vi "Test_firmware_propmt.vi"(8 "WIFI Listo":bool, 11 "ESP32 Listo":bool) -> (2 "Resultado":bool)   [LabVIEW 2025]
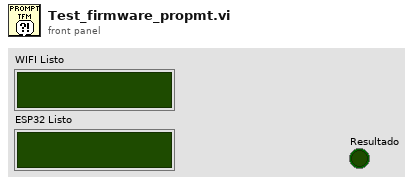
[diagram p1: front panel]
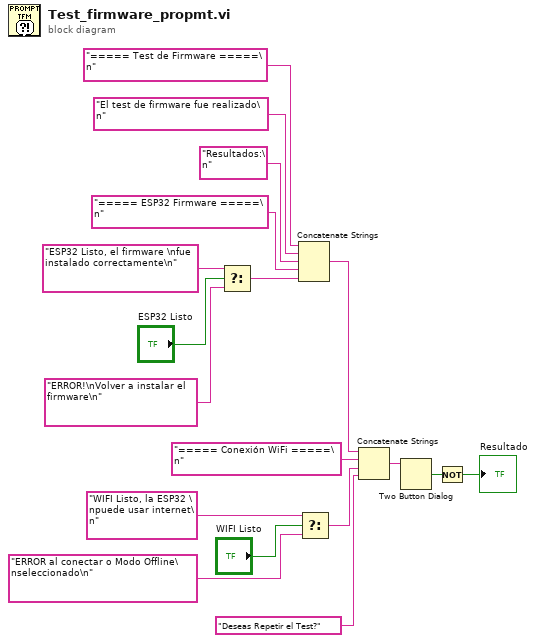
[diagram p0: block diagram]
diagram:
  n1 = Select(t="ESP32 Listo, el firmware \nfue instalado correctamente\n" ("message"), s="ESP32 Listo", f="ERROR!\nVolver a instalar el firmware\n" ("message")) -> (s? t:f=w15:string)
  n2 = Concatenate Strings("===== Test de Firmware =====\n" ("string"), "El test de firmware fue realizado\n" ("string"), "Resultados:\n" ("string"), "===== ESP32 Firmware =====\n" ("string"), w15) -> (w16:string)
  n3 = Select(t="WIFI Listo, la ESP32 \npuede usar internet\n" ("message"), s="WIFI Listo", f="ERROR al conectar o Modo Offline\nseleccionado\n" ("message")) -> (s? t:f=w17:string)
  n4 = Concatenate Strings(w16, "===== Conexión WiFi =====\n" ("string"), w17, "Deseas Repetir el Test?" ("string")) -> (w18:string)
  n5 = Two Button Dialog(message=w18) -> (T button?=w4:bool)  [unwired: 2 in]
  n6 = Not(x=w4) -> (.not. x?=→"Resultado":bool)
